vi "VHMI-recieveSettings.vi"(8 "error in (no error)":errorcluster, 10 "Settings":T1, 11 "VHMI-VNA_Hardware_manager_Interface in":refnum<class "VHMI-VNA_Hardware_manager_Interface.lvclass">) -> (0 "error out":errorcluster, 3 "VHMI-VNA_Hardware_manager_Interface out":refnum<class "VHMI-VNA_Hardware_manager_Interface.lvclass">)   [LabVIEW 2020, in "VHMI-VNA_Hardware_manager_Interface.lvlib" / "VHMI-VNA_Hardware_manager_Interface.lvclass"]
uses:
  VHMI-VNA_Hardware_manager_Interface.lvclass
  classes/vna-drivers/liteVNA/VD-settings_status.ctl
  classes/vna-drivers/liteVNA/VD-LV-LiteVNA.lvclass
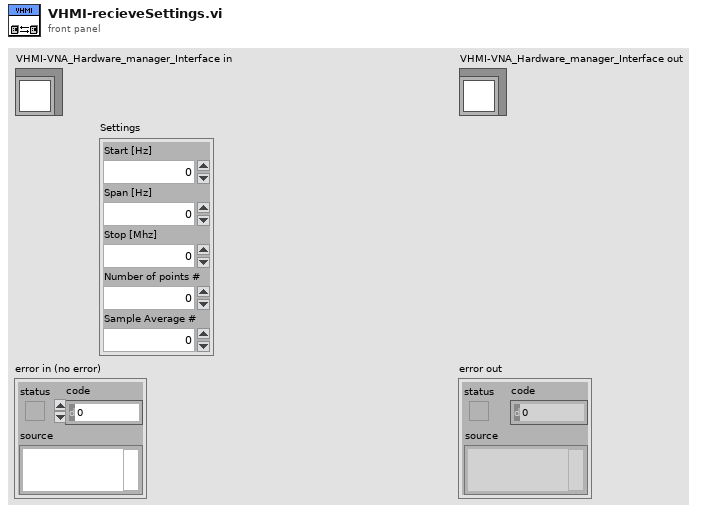
[diagram p1: front panel]
types:
  T1 = typedef "VD-LV-LiteVNA.lvclass/VD-settings_status.ctl" = cluster{"Start [Hz]":u64, "Span [Hz]":u64, "Stop [Mhz]":u64, "Number of points #":u16, "Sample Average #":u16}
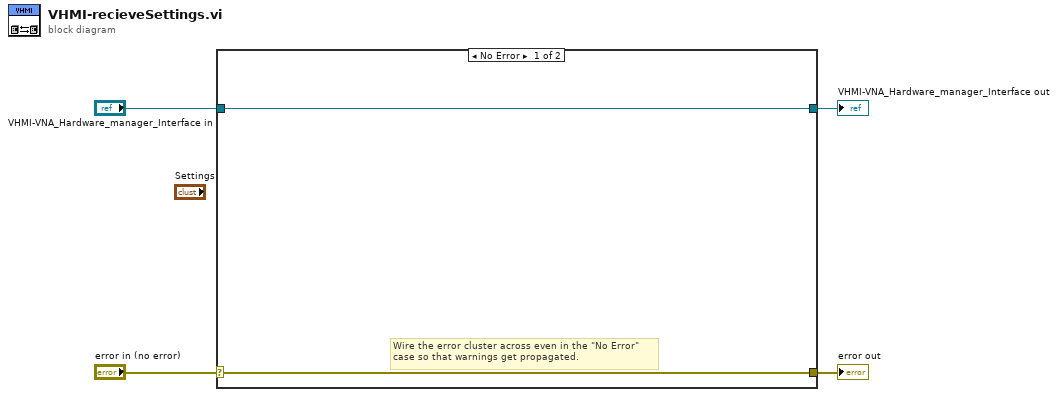
[diagram p0: block diagram]
diagram:
  n1 = case shown="No Error" "error in (no error)" {
    selector: "error in (no error)" -> [w5 w8]
    tunnel: [w5 w8] -> w3
    tunnel: [w6 w7] -> w1
    tunnel: "VHMI-VNA_Hardware_manager_Interface in" -> [w6 w7]
    frame No Error {
      # "Wire the error cluster across even in the \"No Error\"\ncase so that warnings get propagated."
    }
    frame Error {
    }
  }
  "error out" <- w3
  "VHMI-VNA_Hardware_manager_Interface out" <- w1
